vi "Front_Lifter_Function.vi"(4 "Joystick Values":T2) -> (1 "Lifter Status":T1)   [LabVIEW 2014]
panel:
  in  "Lifter Status Def":T1
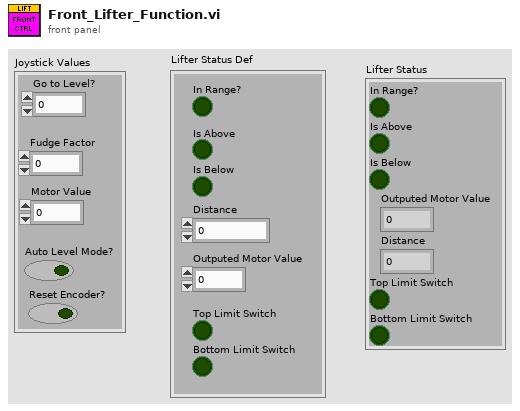
[diagram p1: front panel]
types:
  T1 = cluster{"In Range?":bool, "Is Above":bool, "Is Below":bool, "Outputed Motor Value":dbl, "Distance":dbl, "Top Limit Switch":bool, "Bottom Limit Switch":bool}
  T2 = cluster{"Go to Level?":i32, "Fudge Factor":dbl, "Auto Level Mode?":bool, "Motor Value":dbl, "Reset Encoder?":bool}
  T3 = typedef "WPI_EncoderDevRef.ctl" = cluster{"DevStatus":errorcluster, "EncoderIndex":T4, "CounterIndex":T5, "DistancePerCount":dbl, "Decoding Type":T6}
  T4 = typedef "FPGA_EncoderIdx.ctl" = enum8{"Enc 0", "Enc 1", "Enc 2", "Enc 3", "Enc 4", "Enc 5", "Enc 6", "Enc 7", "Invalid"}
  T5 = typedef "FPGA_CounterCtrSystemIndex.ctl" = enum8{"Ctr 0", "Ctr 1", "Ctr 2", "Ctr 3", "Ctr 4", "Ctr 5", "Ctr 6", "Ctr 7", "Invalid"}
  T6 = typedef "WPI_EncoderType.ctl" = enum16{"1x", "2x", "4x"}
  T7 = typedef "WPI_SwitchDevRef.ctl" = cluster{"DevStatus":errorcluster, "DIO Channel":T8, "Controller":T9, "CntIndex":T5, "Normally Closed":bool}
  T8 = typedef "FPGA_DIOChannel.ctl" = enum8{"DIO 0", "DIO 1", "DIO 2", "DIO 3", "DIO 4", "DIO 5", "DIO 6", "DIO 7", "DIO 8", "DIO 9", "DIO MXP 0", "DIO MXP 1", "DIO MXP 2", "DIO MXP 3", "DIO MXP 4", "DIO MXP 5", "DIO MXP 6", "DIO MXP 7", "DIO MXP 8", "DIO MXP 9", "DIO MXP 10", "DIO MXP 11", "DIO MXP 12", "DIO MXP 13", "DIO MXP 14", "DIO MXP 15", "Invalid"}
  T9 = typedef "FPGA_TypedefDigitalModule.ctl" = enum16{"Controller 1"}
  T10 = typedef "WPI_MotorControlDeviceRef.ctl" = cluster{"DeviceStatus":errorcluster, "Type":T11, "PWM":cluster{"Controller":T9, "PWM Channel":T12, "DeadBand":T13}, "CAN":cluster{"Device Number":u8, "Control Mode":T14, "Semaphore":T15, "Max Vout":dbl, "TalonSRX Control Mode":T16}, "Invert":bool, "TransformRef":T17, "InvTransformRef":T17}
  T11 = typedef "WPI_MotorControlType.ctl" = enum16{"PWM", "CAN", "CANTalonSRX"}
  T12 = typedef "FPGA_DIOPWMChannel.ctl" = enum8{"PWM 0", "PWM 1", "PWM 2", "PWM 3", "PWM 4", "PWM 5", "PWM 6", "PWM 7", "PWM 8", "PWM 9", "PWM MXP 0", "PWM MXP 1", "PWM MXP 2", "PWM MXP 3", "PWM MXP 4", "PWM MXP 5", "PWM MXP 6", "PWM MXP 7", "PWM MXP 8", "PWM MXP 9", "Invalid"}
  T13 = typedef "WPI_PWMDeadband.ctl" = cluster{"Name":string, "maxPositivePwm":i32, "minPositivePwm":i32, "centerPwm":i32, "maxNegativePwm":i32, "minNegativePwm":i32, "angularRange":u16}
  T14 = typedef "WPI_CANJaguar_ControlMode.ctl" = enum8{"Percent VBus", "Current", "Speed", "Position", "Voltage"}
  T15 = typedef "Semaphore RefNum" = refnum<k1>
  T16 = typedef "WPI_CANTalonSRX_APIControlMode.ctl" = enum8{"Percent VBus", "Speed", "Position", "Slave", "Unchanged / Invalid"}
  T17 = typedef "WPI_PWMTransform_ConPane.ctl" = refnum<vi>
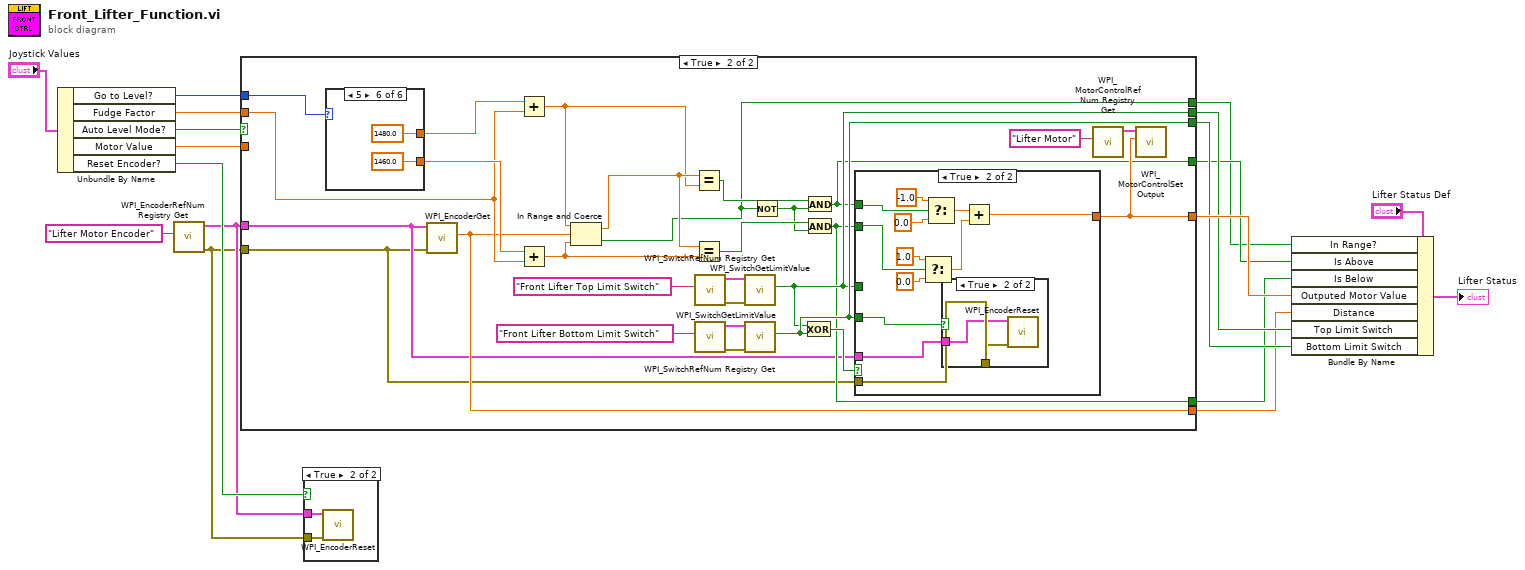
[diagram p0: block diagram]
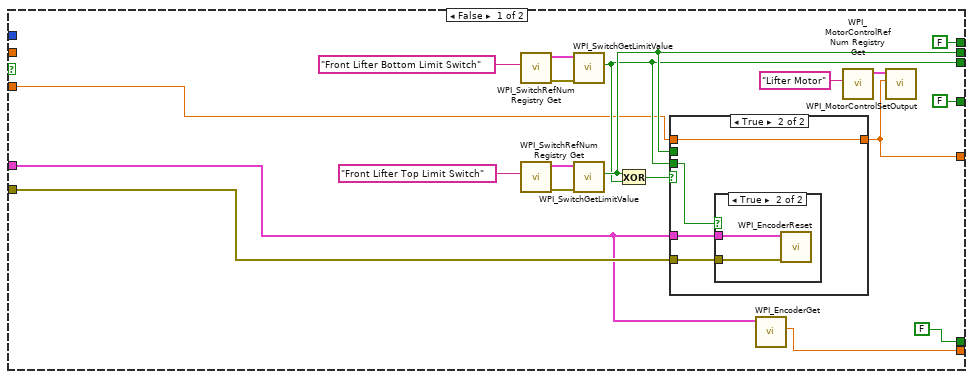
[diagram p3: hidden frame]
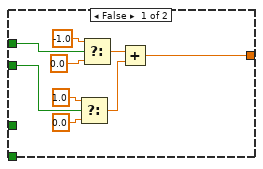
[diagram p6: hidden frame]
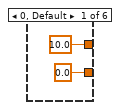
[diagram p8: hidden frame]
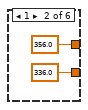
[diagram p9: hidden frame]
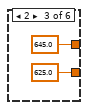
[diagram p10: hidden frame]
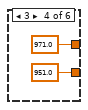
[diagram p11: hidden frame]
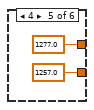
[diagram p12: hidden frame]
diagram:
  n1 = Unbundle By Name("Joystick Values") -> ("Go to Level?"=w17:i32, "Fudge Factor"=w14:dbl, "Auto Level Mode?"=w16:bool, "Motor Value"=w15:dbl, "Reset Encoder?"=w3:bool)
  n2 = call <vilib>:"WPI_EncoderRefNum Registry Get.vi"("refnum name"="Lifter Motor Encoder") -> ("error out"=w1:errorcluster, "EncoderDevRef"=w2:T3)  [unwired: 9 in]
  n3 = case shown="True" w16 {
    tunnel: w15 -> [w21 _]
    tunnel: [w28 w54] -> w11
    tunnel: [w27 w55] -> w10
    tunnel: [w26 w53] -> w12
    tunnel: w17 -> [_ w52]
    tunnel: w14 -> [_ w51]
    tunnel: [w19 w50] -> w9
    tunnel: [FALSE w49] -> w8
    tunnel: [FALSE w48] -> w7
    tunnel: [FALSE w47] -> w6
    tunnel: w2 -> [w20 w46]
    tunnel: w1 -> [w22 w45]
    frame False {
      n4 = call <vilib>:"WPI_SwitchRefNum Registry Get.vi"("refnum name"="Front Lifter Bottom Limit Switch") -> ("error out"=w35:errorcluster, "SwitchDevRef"=w36:T7)  [unwired: 9 in]
      n5 = call <vilib>:"WPI_SwitchRefNum Registry Get.vi"("refnum name"="Front Lifter Top Limit Switch") -> ("error out"=w37:errorcluster, "SwitchDevRef"=w32:T7)  [unwired: 9 in]
      n6 = call <vilib>:"WPI_SwitchGetLimitValue.vi"("error in (no error)"=w35, "SwitchDevRef"=w36) -> ("Switch Pressed"=w27:bool)  [unwired: 7 in, 2 out]
      n7 = call <vilib>:"WPI_SwitchGetLimitValue.vi"("error in (no error)"=w37, "SwitchDevRef"=w32) -> ("Switch Pressed"=w28:bool)  [unwired: 7 in, 2 out]
      n8 = Exclusive Or(1:w27, 2:w28) -> (0:w29:bool)
      n9 = case shown="True" w29 {
        tunnel: w27 -> [_ w40]
        tunnel: w28 -> [_ _]
        tunnel: [w38 w39] -> w26
        tunnel: w21 -> [w38 w39]
        tunnel: w20 -> [_ w42]
        tunnel: w22 -> [_ w41]
        frame False {
        }
        frame True {
          n10 = case shown="True" w40 {
            tunnel: w42 -> [_ w44]
            tunnel: w41 -> [_ w43]
            frame False {
            }
            frame True {
              n11 = call <vilib>:"WPI_EncoderReset.vi"("error in (no error)"=w43, "EncoderDevRef"=w44) -> ()  [unwired: 8 in, 2 out]
            }
          }
        }
      }
      n12 = call <vilib>:"WPI_EncoderGet.vi"("EncoderDevRef"=w20) -> ("Distance"=w19:dbl)  [unwired: 5 in, 5 out]
      n13 = call <vilib>:"WPI_MotorControlRefNum Registry Get.vi"("refnum name"="Lifter Motor") -> ("MotorControlDevRef"=w30:T10)  [unwired: 9 in, 1 out]
      n14 = call <vilib>:"WPI_MotorControlSetOutput.vi"("Output"=w26, "MotorControlDevRef"=w30) -> ()  [unwired: 7 in, 3 out]
    }
    frame True {
      n15 = case shown="5" w52 {
        tunnel: [10.0 ("upper limit") 356.0 ("upper limit") 645.0 ("upper limit") 971.0 ("upper limit") 1277.0 ("upper limit") 1480.0 ("upper limit")] -> w61
        tunnel: [0.0 ("lower Limit") 336.0 ("lower Limit") 625.0 ("lower Limit") 951.0 ("lower Limit") 1257.0 ("lower Limit") 1460.0 ("lower Limit")] -> w60
        frame 0, Default {
        }
        frame 1 {
        }
        frame 2 {
        }
        frame 3 {
        }
        frame 4 {
        }
        frame 5 {
        }
      }
      n16 = call <vilib>:"WPI_EncoderGet.vi"("error in (no error)"=w45, "EncoderDevRef"=w46) -> ("Distance"=w50:dbl)  [unwired: 4 in, 5 out]
      n17 = Add(x=w61, y=w51) -> (x+y=w58:dbl)
      n18 = Add(x=w60, y=w51) -> (x+y=w59:dbl)
      n19 = In Range and Coerce(upper limit=w58, x=w50, lower limit=w59) -> (coerced(x)=w65:dbl, In Range?=w47:bool)
      n20 = Equal?(x=w65, y=w58) -> (x = y?=w56:bool)
      n21 = Equal?(x=w65, y=w59) -> (x = y?=w64:bool)
      n22 = call <vilib>:"WPI_SwitchRefNum Registry Get.vi"("refnum name"="Front Lifter Top Limit Switch") -> ("error out"=w72:errorcluster, "SwitchDevRef"=w71:T7)  [unwired: 9 in]
      n23 = call <vilib>:"WPI_SwitchRefNum Registry Get.vi"("refnum name"="Front Lifter Bottom Limit Switch") -> ("error out"=w69:errorcluster, "SwitchDevRef"=w70:T7)  [unwired: 9 in]
      n24 = call <vilib>:"WPI_SwitchGetLimitValue.vi"("error in (no error)"=w72, "SwitchDevRef"=w71) -> ("Switch Pressed"=w54:bool)  [unwired: 7 in, 2 out]
      n25 = call <vilib>:"WPI_SwitchGetLimitValue.vi"("error in (no error)"=w69, "SwitchDevRef"=w70) -> ("Switch Pressed"=w55:bool)  [unwired: 7 in, 2 out]
      n26 = Not(x=w47) -> (.not. x?=w63:bool)
      n27 = Exclusive Or(1:w55, 2:w54) -> (0:w57:bool)
      n28 = And(x=w56, y=w63) -> (x .and. y?=w48:bool)
      n29 = And(x=w64, y=w63) -> (x .and. y?=w49:bool)
      n30 = case shown="True" w57 {
        tunnel: w48 -> [w74 w83]
        tunnel: w49 -> [w75 w84]
        tunnel: [w73 w82] -> w53
        tunnel: w54 -> [_ _]
        tunnel: w55 -> [_ w92]
        tunnel: w46 -> [_ w93]
        tunnel: w45 -> [_ w91]
        frame False {
          n31 = Select(t=1.0, s=w75, f=0.0) -> (s? t:f=w81:dbl)
          n32 = Select(t=-1.0, s=w74, f=0.0) -> (s? t:f=w80:dbl)
          n33 = Add(x=w80, y=w81) -> (x+y=w73:dbl)
        }
        frame True {
          n34 = Select(t=1.0, s=w84, f=0.0) -> (s? t:f=w90:dbl)
          n35 = Select(t=-1.0, s=w83, f=0.0) -> (s? t:f=w89:dbl)
          n36 = case shown="True" w92 {
            tunnel: w93 -> [_ w95]
            tunnel: w91 -> [_ w94]
            frame False {
            }
            frame True {
              n37 = call <vilib>:"WPI_EncoderReset.vi"("error in (no error)"=w94, "EncoderDevRef"=w95) -> ()  [unwired: 8 in, 2 out]
            }
          }
          n38 = Add(x=w89, y=w90) -> (x+y=w82:dbl)
        }
      }
      n39 = call <vilib>:"WPI_MotorControlRefNum Registry Get.vi"("refnum name"="Lifter Motor") -> ("MotorControlDevRef"=w62:T10)  [unwired: 9 in, 1 out]
      n40 = call <vilib>:"WPI_MotorControlSetOutput.vi"("Output"=w53, "MotorControlDevRef"=w62) -> ()  [unwired: 7 in, 3 out]
    }
  }
  n41 = case shown="True" w3 {
    tunnel: w2 -> [_ w109]
    tunnel: w1 -> [_ w108]
    frame False {
    }
    frame True {
      n42 = call <vilib>:"WPI_EncoderReset.vi"("error in (no error)"=w108, "EncoderDevRef"=w109) -> ()  [unwired: 8 in, 2 out]
    }
  }
  n43 = Bundle By Name(cluster="Lifter Status Def", "In Range?"=w6, "Is Above"=w7, "Is Below"=w8, "Outputed Motor Value"=w12, "Distance"=w9, "Top Limit Switch"=w11, "Bottom Limit Switch"=w10) -> (→"Lifter Status":T1)
